vi "Smart IO Set Led Device Buffer.vi"(8 "error in (no error)":errorcluster, 9 "buffer Data":u32[](array[colorbox]), 11 "deviceIndex":i32=-1) -> (0 "error out":errorcluster)   [LabVIEW 2026, in "MrcLib.lvlib"]
doc: "Update the LED color buffer for the wired device channel or leave device unwired if you choose to update the entire buffer in a single call."
uses:
  MrcLib.lvlib
  Types/MRC Smart IO Mode.ctl
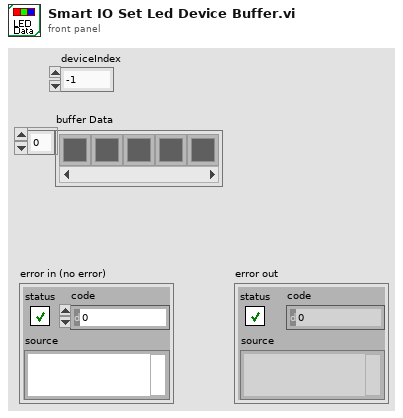
[diagram p1: front panel]
types:
  T1 = typedef "MRC Smart IO Mode.ctl" = i32
  T2 = enum16{"update device span", "update LED buffer", "clear"}
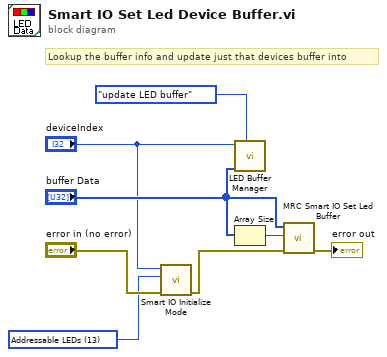
[diagram p0: block diagram]
diagram:
  w1 = T1 13 items=["Digital Input"=0, "Digital Output"=1, "Analog Input"=2, "PWM Input"=3, "PWM Output"=4, "Counter Rising"=5, "Counter Falling"=6, "Addressable LEDs"=13] ("mode")
  # "Lookup the buffer info and update just that devices buffer into"
  n1 = call "Smart IO Initialize Mode.vi"("error in (no error)"="error in (no error)", "mode"=w1, "deviceIndex"="deviceIndex") -> ("error out"=w3:errorcluster)  [unwired: 8 in]
  n2 = call "LED Buffer Manager.vi"("action"=T2."update LED buffer", "Colors"="buffer Data", "deviceIndex"="deviceIndex") -> ()  [unwired: 9 in]
  n3 = Array Size(array="buffer Data") -> (size(s)=w7:i32)
  n4 = call "MRC Smart IO Set Led Buffer.vi"("error in (no error)"=w3, "bufferLength"=w7, "buffer Data"="buffer Data") -> ("error out"=→"error out":errorcluster)  [unwired: 8 in]
